vi "test_Set RIO Resource.vi"(8 "error in (no error)":errorcluster, 11 "TestCase in":refnum<class "FPGA Addon Scripting API Unit Tests.lvclass">) -> (0 "error out":errorcluster, 3 "TestCase out":refnum<class "FPGA Addon Scripting API Unit Tests.lvclass">)   [LabVIEW 2020, in "FPGA Addon Scripting API Unit Tests.lvclass"]
uses:
  FPGA Addon Scripting API Unit Tests.lvclass
  <vilib>/addons/_JKI Toolkits/VI Tester/TestCase.llb/TestCase.lvclass
  FPGA Addon Test Class/FPGA Addon Test Class.lvclass
  APIs/Scripting API/Scripting API.lvlib
  C:/Program Files (x86)/National Instruments/LabVIEW 2020/vi.lib/addons/_JKI Toolkits/VI Tester/TestCase.llb/TestCase.lvclass
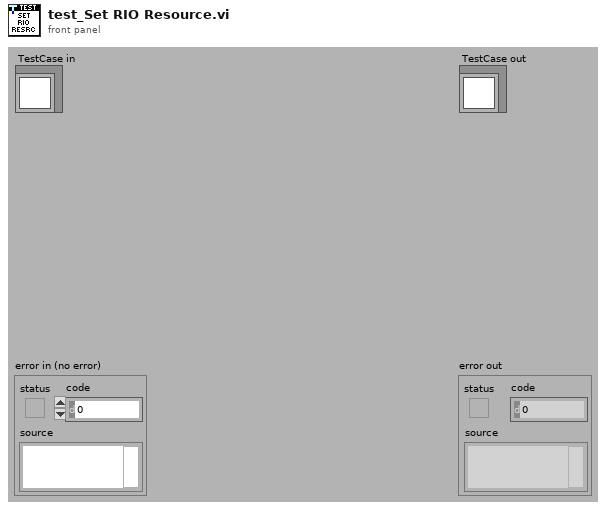
[diagram p1: front panel]
types:
  T1 = typedef "Custom Device API.lvlib/Custom Device Item Ref.ctl" = u64
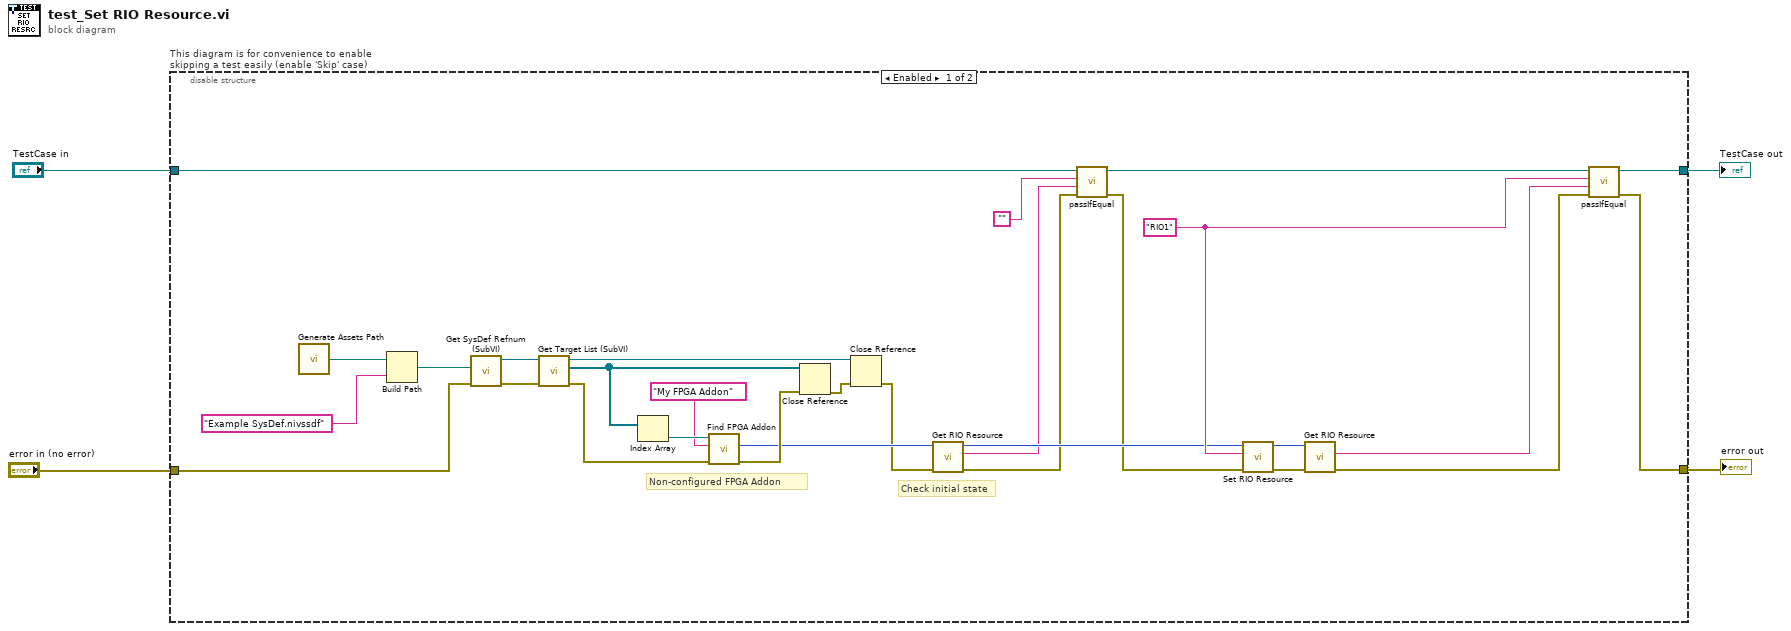
[diagram p0: block diagram]
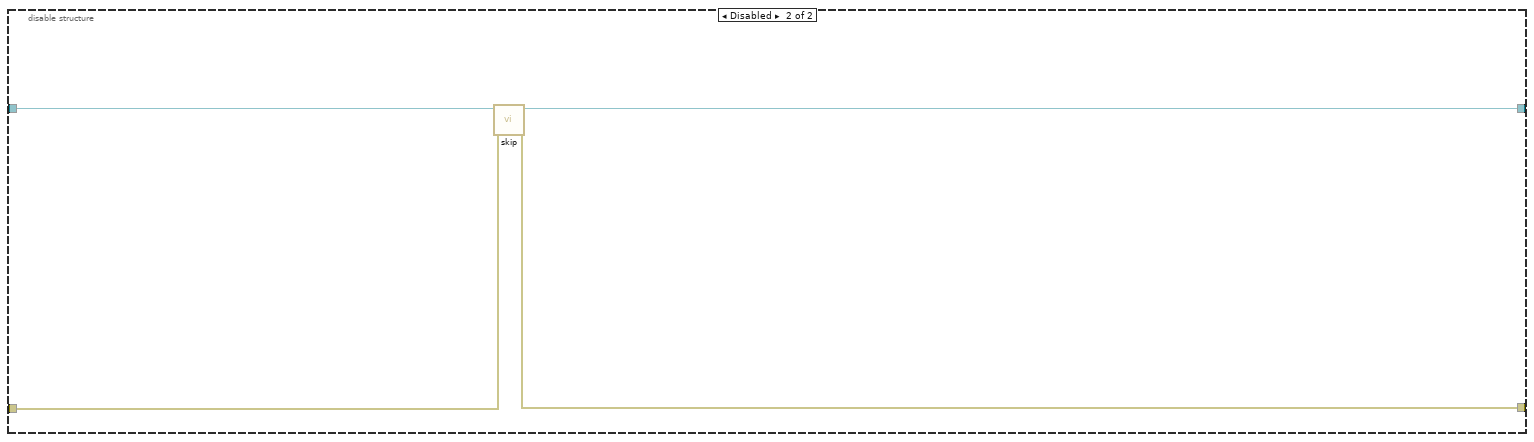
[diagram p2: hidden frame]
diagram:
  n1 = disable-structure "This diagram is for convenience to enable skipping a test easily (enable 'Skip' case)" shown="Enabled" {
    disable-tunnel: "TestCase in" -> [w10 w37]
    disable-tunnel: [w19 w35] -> w1
    disable-tunnel: [w20 w36] -> w3
    disable-tunnel: "error in (no error)" -> [w29 w34]
    frame Enabled {
      w14 = "RIO1" ("RIO resource")
      # "Check initial state"
      # "Non-configured FPGA Addon"
      n2 = call "Generate Assets Path.vi"() -> ("Assets path"=w33:path)
      n3 = Build Path(base path=w33, name or relative path="Example SysDef.nivssdf") -> (appended path=w31:path)
      n4 = call "Get SysDef Refnum (SubVI).vi"("error in (no error)"=w29, "System Definition path"=w31) -> ("error out"=w28:errorcluster, "SysDef Refnum out"=w30:refnum<k24>)  [unwired: 8 in]
      n5 = call "Get Target List (SubVI).vi"("error in (no error)"=w28, "SysDef Refnum in"=w30) -> ("error out"=w23:errorcluster, "Target List Refnums"=w27:refnum<k24>[], "SysDef Refnum out"=w26:refnum<k24>)  [unwired: 7 in]
      n6 = Index Array(array=w27) -> (element=w24:refnum<k24>)  [unwired: 1 in]
      n7 = call "Find FPGA Addon.vi"("error in"=w23, "FPGA addon name"="My FPGA Addon", "target in"=w24) -> ("error out"=w21:errorcluster, "FPGA addon refnum out"=w13:T1)  [unwired: 5 in, 2 out]
      n8 = Close Reference(reference=w27, error in (no error)=w21) -> (error out=w25:errorcluster)
      n9 = Close Reference(reference=w26, error in (no error)=w25) -> (error out=w12:errorcluster)
      n10 = call "Get RIO Resource.vi"("error in"=w12, "FPGA addon refnum in"=w13) -> ("error out"=w8:errorcluster, "RIO resource"=w6:string, "FPGA addon refnum out"=w11:T1)  [unwired: 7 in]
      n11 = call-dynamic "passIfEqual.vi"("error in (no error)"=w8, "y"=w6, "x"="", "TestCase in"=w10) -> ("error out"=w7:errorcluster, "TestCase out"=w9:refnum<class "FPGA Addon Scripting API Unit Tests.lvclass">)  [unwired: 6 in]
      n12 = call "Set RIO Resource.vi"("error in"=w7, "RIO resource in"=w14, "FPGA addon refnum in"=w11) -> ("error out"=w15:errorcluster, "FPGA addon refnum out"=w16:T1)  [unwired: 7 in]
      n13 = call "Get RIO Resource.vi"("error in"=w15, "FPGA addon refnum in"=w16) -> ("error out"=w18:errorcluster, "RIO resource"=w17:string)  [unwired: 7 in, 1 out]
      n14 = call-dynamic "passIfEqual.vi"("error in (no error)"=w18, "y"=w17, "x"=w14, "TestCase in"=w9) -> ("error out"=w20:errorcluster, "TestCase out"=w19:refnum<class "FPGA Addon Scripting API Unit Tests.lvclass">)  [unwired: 6 in]
    }
    frame Disabled {
      # "skip test result while test is under development"
      n15 = call <vilib>:"skip.vi"("error in (no error)"=w34, "TestCase in"=w37) -> ("error out"=w36:errorcluster, "TestCase out"=w35:refnum<class "FPGA Addon Scripting API Unit Tests.lvclass">)  [unwired: 8 in]
    }
  }
  "error out" <- w3
  "TestCase out" <- w1
